vi "Enqueue Multiple Messages.vi"(8 "error in (no error)":errorcluster, 10 "queue in":refnum<queue>, 11 "Message in":refnum<class "Message.lvclass">[](array[class])) -> (0 "error out":errorcluster, 2 "queue out":refnum<queue>)   [LabVIEW 2021, in "Architecture.lvlib" / "Message.lvclass"]
doc: "Enqueue several messages in a message local queue"
uses:
  Message.lvclass
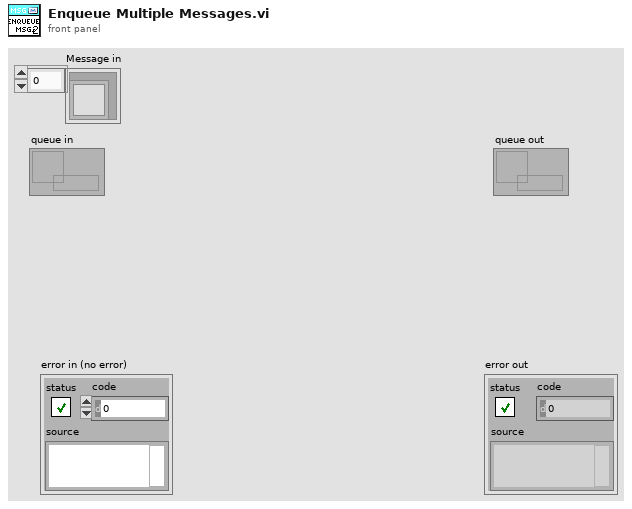
[diagram p1: front panel]
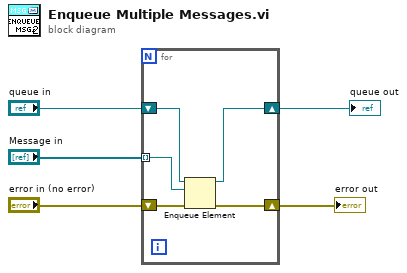
[diagram p0: block diagram]
diagram:
  n1 = for {
    tunnel: "Message in" -> [w7] mode=indexing
    shift-right: [w9] -> w4
    shift-left: "error in (no error)" -> [w10]
    shift-right: [w6] -> w1
    shift-left: "queue in" -> [w8]
    n2 = Enqueue Element(queue=w8, element=w7, error in (no error)=w10) -> (queue out=w6:refnum<queue>, error out=w9:errorcluster)  [unwired: 1 in, 1 out]
  }
  "error out" <- w4
  "queue out" <- w1
